vi "Open Base System Definition.vi"(8 "error in (no error)":errorcluster) -> (0 "error out":errorcluster, 2 "Routing and Faulting Custom Device Ref":T1 format="%.0x", 3 "SystemDefinition":refnum<k24>)   [LabVIEW 2019, in "Routing and Faulting Scripting System Tests.lvclass"]
uses:
  Routing and Faulting Scripting System Tests.lvclass
  <vilib>/NI/VeriStand Custom Device Testing Tools/VeriStandTestUtilities/VeriStandTestUtilities.lvlib
  <userlib>/_OpenG.lib/file/file.llb/Append Path to Root if Relative - Scalar__ogtk.vi
  NationalInstruments.VeriStand.SystemDefinitionAPI
  Routing and Faulting Scripting.lvlib
  <vilib>/NI VeriStand/Custom Device API/Custom Device Item Ref.ctl
  <vilib>/NI VeriStand/Custom Device API/Custom Device API.lvlib
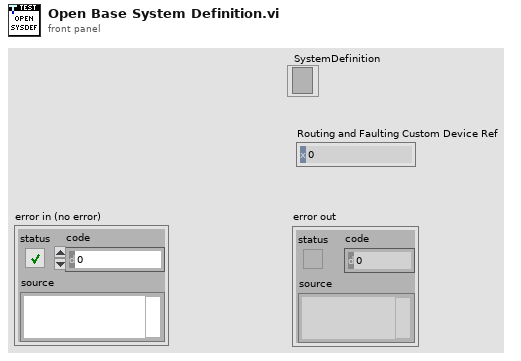
[diagram p1: front panel]
types:
  T1 = typedef "Custom Device API.lvlib/Custom Device Item Ref.ctl" = u64
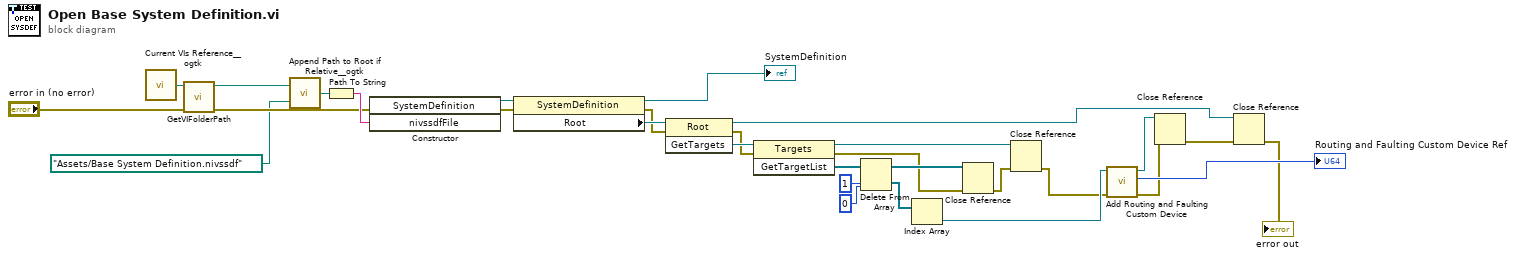
[diagram p0: block diagram]
diagram:
  n1 = call <userlib>:"Current VIs Reference__ogtk.vi"() -> ("Current VI's reference"=w8:refnum<vi>)  [unwired: 5 in]
  n2 = call <vilib>:"GetVIFolderPath.vi"("error in (no error)"="error in (no error)", "VI Reference in"=w8) -> ("error out"=w12:errorcluster, "VI Folder Path out"=w9:path)  [unwired: 8 in]
  n3 = call-poly <userlib>:"Append Path to Root if Relative__ogtk.vi"("Absolute or Relative Path"=path "Assets/Base System Definition.nivssdf", "Root Path"=w9) -> ("Absolute or Appended Path"=w11:path)
  n4 = Path To String(path=w11) -> (string=w14:string)
  n5 = constructor class="SystemDefinition"(error in=w12, "nivssdfFile"=w14) -> (reference out=w15:refnum<k24>, error out=w13:errorcluster)  [unwired: 2 in, 2 out]
  n6 = property class="SystemDefinition"(reference=w15, error in=w13) -> (reference out=→"SystemDefinition":refnum<k24>, error out=w16:errorcluster, "Root"=w17:refnum<k24>)
  n7 = invoke class="Root" method="GetTargets"(reference=w17, error in=w16) -> (reference out=w1:refnum<k24>, error out=w18:errorcluster, "GetTargets"=w19:refnum<k24>)  [unwired: 1 in]
  n8 = invoke class="Targets" method="GetTargetList"(reference=w19, error in=w18) -> (reference out=w26:refnum<k24>, error out=w23:errorcluster, "GetTargetList"=w20:refnum<k24>[])  [unwired: 1 in]
  n9 = Delete From Array(array=w20, length=1, index=0) -> (deleted portion=w27:refnum<k24>[], array with subset deleted=w24:refnum<k24>[])
  n10 = Index Array(array=w27) -> (element=w30:refnum<k24>)  [unwired: 1 in]
  n11 = Close Reference(reference=w24, error in (no error)=w23) -> (error out=w25:errorcluster)
  n12 = Close Reference(reference=w26, error in (no error)=w25) -> (error out=w29:errorcluster)
  n13 = call "Add Routing and Faulting Custom Device.vi"("error in"=w29, "target in"=w30) -> ("error out"=w6:errorcluster, "routing and faulting custom device"=→"Routing and Faulting Custom Device Ref":T1, "target out"=w5:refnum<k24>)  [unwired: 7 in]
  n14 = Close Reference(reference=w5, error in (no error)=w6) -> (error out=w3:errorcluster)
  n15 = Close Reference(reference=w1, error in (no error)=w3) -> (error out=→"error out":errorcluster)
